vi "RgbaToU32_2D.vi"(11 "Rgba":T1[][](array[typedef])) -> (3 "U32":u32[][](array[numeric]))   [LabVIEW 2024, in "OpenLvVision_Image.lvlib" / "DataAccess.lvlib"]
doc: "Convert an color cluster into an number"
uses:
  DataAccess.lvlib
  TypeDef/RgbaU32.ctl
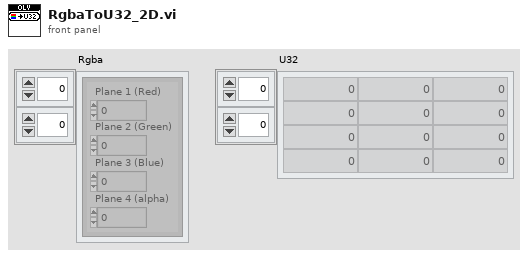
[diagram p1: front panel]
types:
  T1 = typedef "OpenLvVision_Image.lvlib/DataAccess.lvlib/RgbaU32.ctl" = cluster{"Plane 1 (Red)":u8, "Plane 2 (Green)":u8, "Plane 3 (Blue)":u8, "Plane 4 (alpha)":u8}
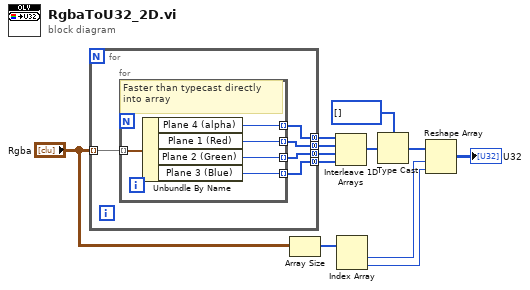
[diagram p0: block diagram]
diagram:
  n1 = for {
    tunnel: [w17] -> w12 mode=concatenating
    tunnel: [w16] -> w11 mode=concatenating
    tunnel: [w15] -> w10 mode=concatenating
    tunnel: [w14] -> w9 mode=concatenating
    tunnel: "Rgba" -> [w13] mode=indexing
    n2 = for {
      tunnel: [w22] -> w17 mode=indexing
      tunnel: [w21] -> w15 mode=indexing
      tunnel: [w20] -> w16 mode=indexing
      tunnel: [w19] -> w14 mode=indexing
      tunnel: w13 -> [w18] mode=indexing
      # "Faster than typecast directly into array"
      n3 = Unbundle By Name(w18) -> ("Plane 4 (alpha)"=w22:u8, "Plane 1 (Red)"=w21:u8, "Plane 2 (Green)"=w20:u8, "Plane 3 (Blue)"=w19:u8)
    }
  }
  n4 = Array Size(array="Rgba") -> (size(s)=w3:i32[])
  n5 = Interleave 1D Arrays(w12, w10, w11, w9) -> (w8:u8[])
  n6 = Index Array(array=w3) -> (element #1=w2:i32, element #2=w1:i32)  [unwired: 2 in]
  n7 = Type Cast(type=u32[] [], x=w8) -> (*(type *) &x=w6:u32[])
  n8 = Reshape Array(w6, w2, w1) -> (→"U32":u32[][])
